vi "AddDependenciesOfLibrary.vi"(8 "error in (no error)":errorcluster, 9 "LibraryName":string="ModuleA", 10 "Project Path":path=path "E:/sw-deps-monitor/Source/BuildSpecs/Modules/ModuleA.lvproj", 11 "Config Refnum in":T1) -> (0 "error out":errorcluster, 1 "Indirect ActualDependencies":string[](array[string]), 2 "Direct ActualDependencies":string[](array[string]), 3 "Config Refnum out":T1)   [LabVIEW 2019, in "Hawkeye.lvlib"]
uses:
  Hawkeye.lvlib
  <vilib>/Utility/config.llb/Config Data RefNum.ctl
  <vilib>/Utility/config.llb/Write Key (String).vi
  <vilib>/Utility/config.llb/NI_LVConfig.lvlib
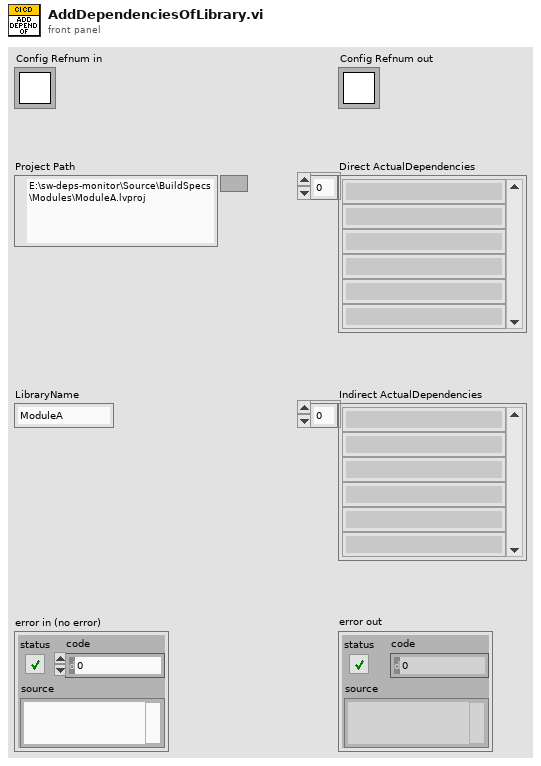
[diagram p1: front panel]
types:
  T1 = typedef "NI_LVConfig.lvlib/Config Data RefNum.ctl" = refnum<k1>
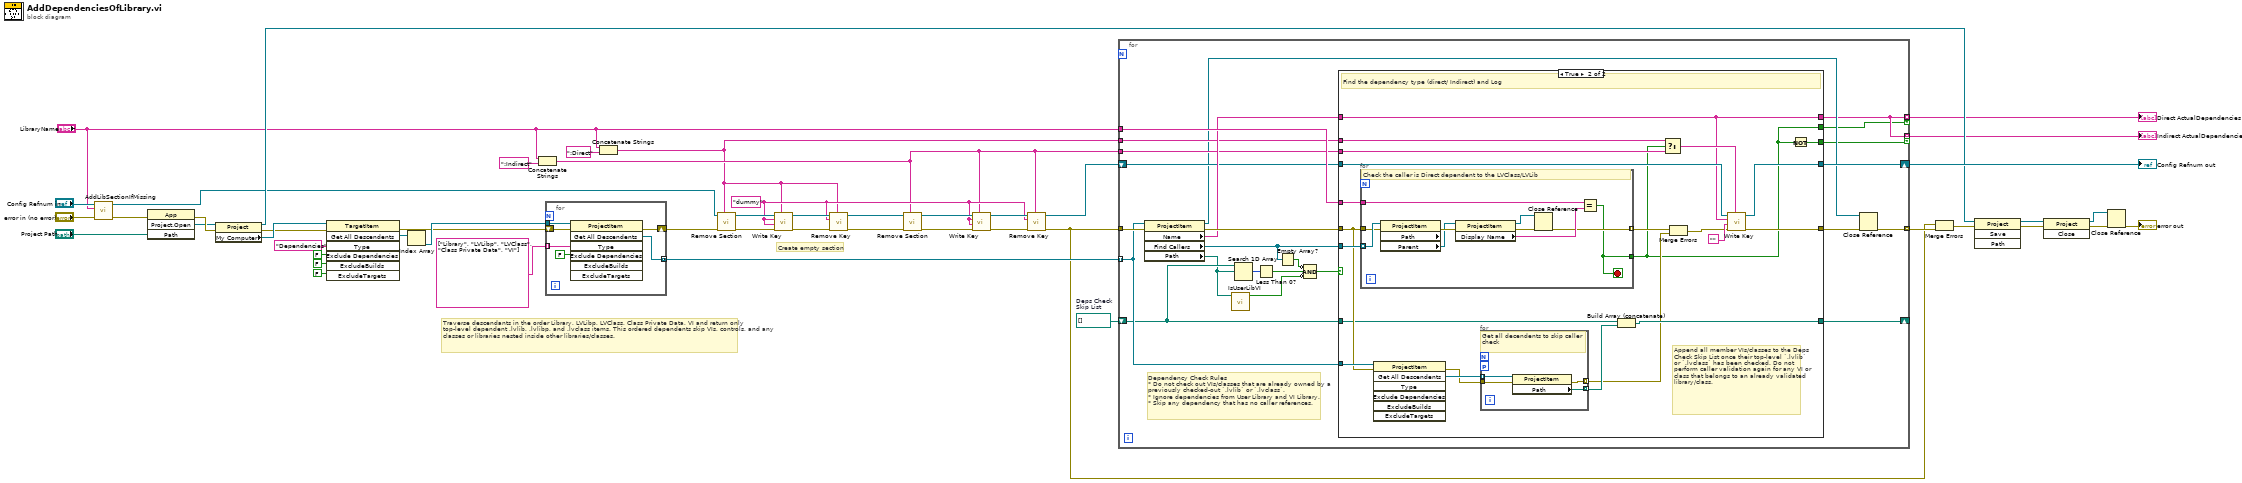
[diagram p0: block diagram]
diagram:
  w1 = path[] []  # Deps Check  Skip List
  w10 = "dummy" ("key")
  # "Traverse descendants in the order Library, LVLibp, LVClass, Class Private Data, VI and return only top-level dependent .lvlib, .lvlibp, and .lvclass items. This ordered dependents skip VIs, controls, and any classes or libraries nested inside other libraries/classes."
  # "Create empty section"
  n1 = call "AddLibSectionIfMissing.vi"("error in (no error)"="error in (no error)", "LibraryName"="LibraryName", "Config Refnum in"="Config Refnum in") -> ("error out"=w29:errorcluster, "Config Refnum out"=w26:T1)  [unwired: 7 in]
  n2 = invoke class="App" method="Project.Open"(error in=w29, "Path"="Project Path") -> (error out=w48:errorcluster, "Project:Open"=w47:refnum<vi>)  [unwired: 2 in, 2 out]
  n3 = property class="Project"(reference=w47, error in=w48) -> (reference out=w34:refnum<vi>, error out=w37:errorcluster, "My Computer"=w41:refnum<vi>)
  n4 = invoke class="TargetItem" method="Get All Descendents"(reference=w41, error in=w37, "Type"="Dependencies", "Exclude Dependencies"=FALSE ("ExcludeDependencies"), "ExcludeBuilds"=FALSE, "ExcludeTargets"=FALSE) -> (error out=w36:errorcluster, "All Descendents"=w39:refnum<vi>[])  [unwired: 1 in, 5 out]
  n5 = Index Array(array=w39) -> (element=w38:refnum<vi>)  [unwired: 1 in]
  n6 = Concatenate Strings("LibraryName", ":Indirect" ("Type")) -> (w9:string)
  n7 = for {
    tunnel: w38 -> [w54]
    tunnel: [w51] -> w31 mode=concatenating
    shift-right: [w52] -> w32
    shift-left: w36 -> [w53]
    tunnel: string[] ["Library", "LVLibp", "LVClass", "Class Private Data", "VI"] ("Type") -> [w50] mode=indexing
    n8 = invoke class="ProjectItem" method="Get All Descendents"(reference=w54, error in=w53, "Type"=w50, "Exclude Dependencies"=FALSE ("ExcludeDependencies")) -> (error out=w52:errorcluster, "All Descendents"=w51:refnum<vi>[])  [unwired: 3 in, 5 out]
  }
  n9 = Concatenate Strings("LibraryName", ":Direct" ("Type")) -> (w6:string)
  n10 = call <vilib>:"Remove Section.vi"("section"=w6, "error in (no error)"=w32, "refnum"=w26) -> ("error out"=w25:errorcluster, "refnum out"=w24:T1)  [unwired: 6 in, 1 out]
  n11 = call-poly <vilib>:"Write Key.vi"("section"=w6, "error in (no error)"=w25, "value"=w10, "key"=w10, "refnum"=w24) -> ("error out"=w23:errorcluster, "refnum out"=w22:T1)  [unwired: 4 in, 1 out]
  n12 = call <vilib>:"Remove Key.vi"("section"=w6, "error in (no error)"=w23, "key"=w10, "refnum"=w22) -> ("error out"=w14:errorcluster, "refnum out"=w11:T1)  [unwired: 5 in, 1 out]
  n13 = call <vilib>:"Remove Section.vi"("section"=w9, "error in (no error)"=w14, "refnum"=w11) -> ("error out"=w13:errorcluster, "refnum out"=w16:T1)  [unwired: 6 in, 1 out]
  n14 = call-poly <vilib>:"Write Key.vi"("section"=w9, "error in (no error)"=w13, "value"=w10, "key"=w10, "refnum"=w16) -> ("error out"=w17:errorcluster, "refnum out"=w18:T1)  [unwired: 4 in, 1 out]
  n15 = call <vilib>:"Remove Key.vi"("section"=w9, "error in (no error)"=w17, "key"=w10, "refnum"=w18) -> ("error out"=w15:errorcluster, "refnum out"=w12:T1)  [unwired: 5 in, 1 out]
  n16 = for {
    tunnel: w15 -> [w79]
    tunnel: w31 -> [w75] mode=indexing
    tunnel: "LibraryName" -> [w78]
    tunnel: [w62] -> w46 mode=indexing
    shift-right: [w77] -> _
    shift-left: w1 -> [w73]
    tunnel: w6 -> [w66]
    tunnel: w9 -> [w65]
    shift-right: [w63] -> w45
    shift-left: w12 -> [w64]
    tunnel: [w60] -> w27 mode=indexing if=w59
    tunnel: [w60] -> w7 mode=indexing if=w58
    # "Dependency Check Rules\n* Do not check out VIs/classes that are already owned by a previously checked-out `.lvlib` or `.lvclass`.\n* Ignore dependencies from User Library and VI Library.\n* Skip any dependency that has no caller references."
    n17 = property class="ProjectItem"(reference=w75, error in=w79) -> (reference out=w61:refnum<vi>, error out=w76:errorcluster, "Name"=w72:string, "Find Callers"=w57:refnum<vi>[], "Path"=w71:path)
    n18 = call "IsUserLibVI.vi"("ItemPath"=w71) -> ("IsUserLibVI?"=w69:bool)  [unwired: 10 in]
    n19 = Search 1D Array(1D array=w73, element=w71) -> (index of element=w68:i32)  [unwired: 1 in]
    n20 = Less Than 0?(x=w68) -> (x < 0?=w70:bool)
    n21 = Empty Array?(array=w57) -> (empty?=w56:bool)
    n22 = Compound Arithmetic op=AND(invert w56, w70, invert w69) -> (w67:bool)
    n23 = case shown="True" w67 {
      tunnel: w57 -> [_ w104]
      tunnel: w78 -> [_ w103]
      tunnel: [w82 w101] -> w77
      tunnel: w73 -> [w82 w94]
      tunnel: w76 -> [w81 w95]
      tunnel: w75 -> [_ w99]
      tunnel: [w81 w91] -> w74
      tunnel: w72 -> [_ w84]
      tunnel: w66 -> [_ w90]
      tunnel: w65 -> [_ w89]
      tunnel: w64 -> [w80 w87]
      tunnel: [w80 w86] -> w63
      tunnel: [_ w84] -> w60
      tunnel: [_ w85] -> w59
      tunnel: [_ w83] -> w58
      frame False {
      }
      frame True {
        # "Append all member VIs/classes to the Deps Check Skip List once their top-level `.lvlib` or `.lvclass` has been checked. Do not perform caller validation again for any VI or class that belongs to an already validated library/class."
        # "Find the dependency type (direct/ Indirect) and Log"
        n24 = for {
          tunnel: w104 -> [w118] mode=indexing
          tunnel: w103 -> [w113]
          tunnel: [w109] -> w85
          tunnel: [w112] -> w97 mode=indexing
          tunnel: w95 -> [w115]
          stop <- w109 stop-if-true
          # "Check the caller is Direct dependent to the LVClass/LVLib"
          n25 = property class="ProjectItem" props=["Path", "Parent"](reference=w118, error in=w115) -> (error out=w114:errorcluster, "Parent"=w110:refnum<vi>)  [unwired: 2 out]
          n26 = property class="ProjectItem"(reference=w110, error in=w114) -> (reference out=w111:refnum<vi>, error out=w116:errorcluster, "Display Name"=w117:string)
          n27 = Close Reference(reference=w111, error in (no error)=w116) -> (error out=w112:errorcluster)
          n28 = Equal?(x=w113, y=w117) -> (x = y?=w109:bool)
        }
        n29 = invoke class="ProjectItem" method="Get All Descendents"(reference=w99, error in=w95) -> (error out=w98:errorcluster, "All Descendents"=w100:refnum<vi>[])  [unwired: 5 in, 5 out]
        n30 = for {
          tunnel: w100 -> [w108] mode=indexing
          tunnel: [w107] -> w102 mode=indexing
          tunnel: w98 -> [w106]
          tunnel: [w105] -> w96 mode=indexing
          workers-P: _ -> [_]
          # "Get all decendents to skip caller check"
          n31 = property class="ProjectItem"(reference=w108, error in=w106) -> (error out=w105:errorcluster, "Path"=w107:path)  [unwired: 1 out]
        }
        n32 = Build Array (concatenate)(w94, w102) -> (w101:path[])
        n33 = Select(t=w90, s=w85, f=w89) -> (s? t:f=w88:string)
        n34 = Merge Errors(w97, w96) -> (w92:errorcluster)
        n35 = call-poly <vilib>:"Write Key.vi"("section"=w88, "error in (no error)"=w92, "value"="", "key"=w84, "refnum"=w87) -> ("error out"=w91:errorcluster, "refnum out"=w86:T1)  [unwired: 4 in, 1 out]
        n36 = Not(x=w85) -> (.not. x?=w83:bool)
      }
    }
    n37 = Close Reference(reference=w61, error in (no error)=w74) -> (error out=w62:errorcluster)
  }
  "Config Refnum out" <- w45
  "Direct ActualDependencies" <- w27
  "Indirect ActualDependencies" <- w7
  n38 = Merge Errors(w15, w46) -> (w35:errorcluster)
  n39 = invoke class="Project" method="Save"(reference=w34, error in=w35) -> (reference out=w5:refnum<vi>, error out=w3:errorcluster)  [unwired: 2 in, 2 out]
  n40 = invoke class="Project" method="Close"(reference=w5, error in=w3) -> (reference out=w4:refnum<vi>, error out=w2:errorcluster)  [unwired: 1 in, 1 out]
  n41 = Close Reference(reference=w4, error in (no error)=w2) -> (error out=→"error out":errorcluster)
